vi "JSON Editor.vi"() -> ()   [LabVIEW 2024]
uses:
  WebView_class/Editor Mode--enum.ctl
  WebView.JSONEditor_class/WebView.JSONEditor.lvclass/WebView.JSONEditor.ctl
  WebView.JSONEditor_class/properties/Get JSONEditor Events.vi
  WebView.JSONEditor_class/WebView.JSONEditor.lvclass
  <vilib>/JDP Science/JSONtext/JSONtext.lvlib
  <vilib>/sklein/WebView2/Libs/Microsoft.Web.WebView2.WinForms.dll
panel:
  in  "Mode":T1
  out "Node Path":string
  out "Error Out":errorcluster
  in  "Expand all?":bool
  in  "System Load Button":bool
  in  "Stop":bool
  in  "Tab Control":enum32{"JSON", "JSON Schema"}(tab)
  in  "JSON (transparent)":string
  in  "JSON Schema":string
  in  "WebView2 Control in":refnum<k24>(container)
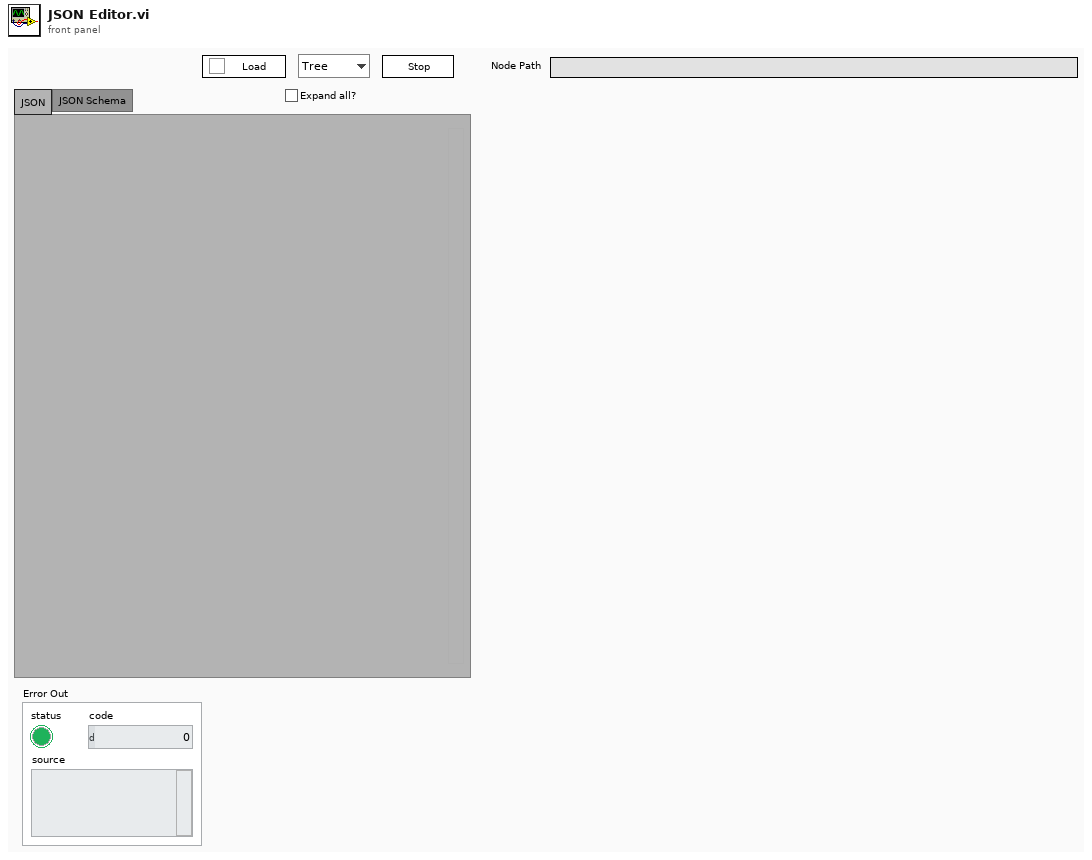
[diagram p1: front panel]
types:
  T1 = typedef "WebView.JSONEditor.lvclass/Editor Mode--enum.ctl" = enum16{"Tree", "View", "Form", "Code", "Text"}
  T2 = typedef "WebView.JSONEditor.lvclass/JSONEditor Events.ctl" = cluster{"JSON Updated":refnum<user-event>, "Selected Node Path":refnum<user-event>}
  T3 = typedef "WebView.JSONEditor.lvclass/Seleced Node Path Event Data--string.ctl" = string
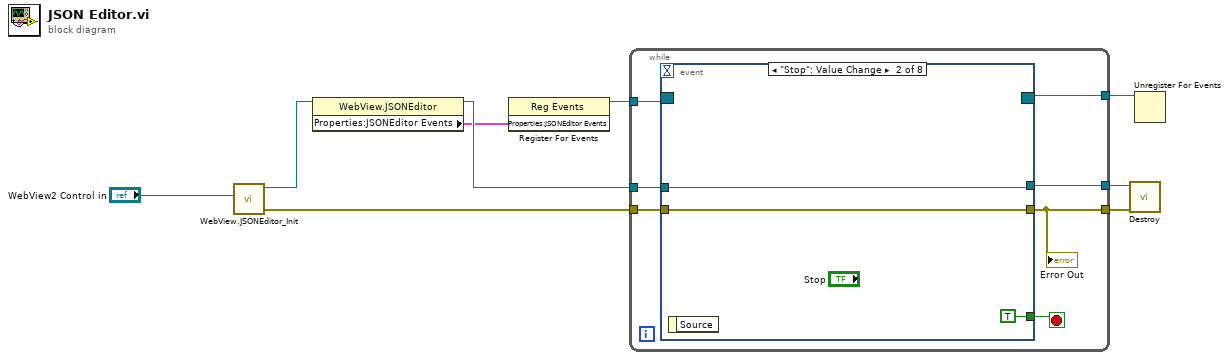
[diagram p0: block diagram]
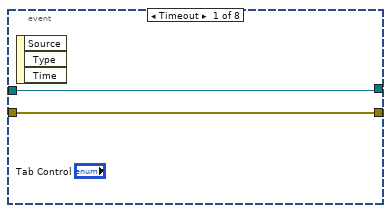
[diagram p2: hidden frame]
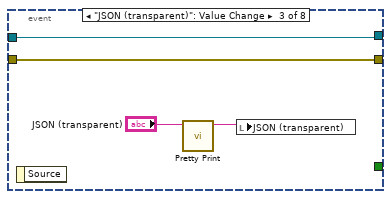
[diagram p3: hidden frame]
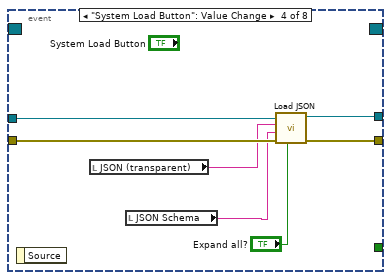
[diagram p4: hidden frame]
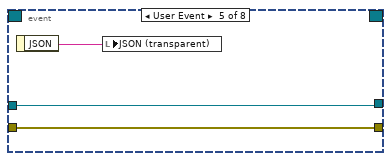
[diagram p5: hidden frame]
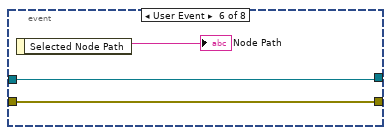
[diagram p6: hidden frame]
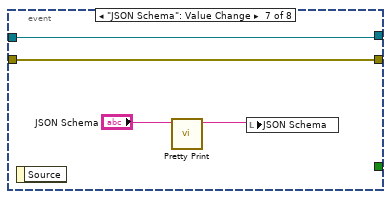
[diagram p7: hidden frame]
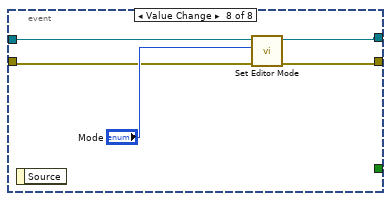
[diagram p8: hidden frame]
diagram:
  n1 = call "WebView.JSONEditor_Init.vi"("WebView2 Control in"="WebView2 Control in") -> ("Error Out"=w7:errorcluster, "WebView.JSONEditor out"=w8:refnum<class "WebView.JSONEditor.lvclass">)  [unwired: 9 in]
  n2 = property class="WebView.JSONEditor"(reference=w8) -> (reference out=w4:refnum<class "WebView.JSONEditor.lvclass">, "Properties:JSONEditor Events"=w2:T2)  [unwired: 1 in, 1 out]
  n3 = register-events(w2) -> (reference out=w3:refnum<event-registration>)  [unwired: 2 in, 1 out]
  n4 = while {
    tunnel: w4 -> [w16]
    tunnel: w7 -> [w15]
    tunnel: [w12] -> w6
    tunnel: [w14] -> w5
    tunnel: w3 -> [w11]
    tunnel: [w10] -> w1
    stop <- w13 stop-if-true
    n5 = event shown="[1] \"Stop\": Value Change" {
      selector: w11 -> [_ _ _ _ _ _ _ _]
      dyn-events: [_ _ _ _ _ _ _ _] -> w10
      timeout: _ -> [_ _ _ _ _ _ _ _]
      tunnel: w16 -> [w18 w19 w23 w31 w34 w37 w40 w46]
      tunnel: w15 -> [w17 w20 w22 w30 w35 w38 w39 w44]
      tunnel: [w17 w20 w22 w29 w35 w38 w39 w43] -> w12
      tunnel: [w18 w19 w23 w28 w34 w37 w40 w47] -> w14
      tunnel: [_ TRUE _ _ _ _ _ _] -> w13
      event Timeout {
        n6 = event-data() -> ()  [unwired: 1 in, 3 out]
      }
      event "Stop": Value Change {
        n7 = event-data() -> ()  [unwired: 1 in, 1 out]
      }
      event "JSON (transparent)": Value Change {
        n8 = event-data() -> ()  [unwired: 1 in, 1 out]
        n9 = call <vilib>:"Pretty Print.vi"("JSON"="JSON (transparent)") -> ("<JSON>"=w24:string)  [unwired: 8 in, 2 out]
        n10 = local write "JSON (transparent)"(w24) -> ()
      }
      event "System Load Button": Value Change {
        n11 = event-data() -> ()  [unwired: 1 in, 1 out]
        n12 = local read "JSON (transparent)"() -> (w27:string)
        n13 = local read "JSON Schema"() -> (w26:string)
        n14 = call "Load JSON.vi"("Expand all?"="Expand all?", "Error In"=w30, "JSON Schema in"=w26, "<JSON> in"=w27, "WebView.JSONEditor in"=w31) -> ("Error Out"=w29:errorcluster, "WebView.JSONEditor out"=w28:refnum<class "WebView.JSONEditor.lvclass">)  [unwired: 5 in]
      }
      event User Event {
        n15 = event-data() -> ("JSON"=w33:string)  [unwired: 1 in]
        n16 = local write "JSON (transparent)"(w33) -> ()
      }
      event User Event {
        n17 = event-data() -> ("Selected Node Path"=→"Node Path":T3)  [unwired: 1 in]
      }
      event "JSON Schema": Value Change {
        n18 = event-data() -> ()  [unwired: 1 in, 1 out]
        n19 = call <vilib>:"Pretty Print.vi"("JSON"="JSON Schema") -> ("<JSON>"=w41:string)  [unwired: 8 in, 2 out]
        n20 = local write "JSON Schema"(w41) -> ()
      }
      event Value Change {
        n21 = event-data() -> ()  [unwired: 1 in, 1 out]
        n22 = call-dynamic "Set Editor Mode.vi"("Error In"=w44, "Mode in"="Mode", "object in"=w46) -> ("Error Out"=w43:errorcluster, "object out"=w47:refnum<class "WebView.JSONEditor.lvclass">)  [unwired: 7 in]
      }
    }
    "Error Out" <- w12
  }
  n23 = call-dynamic "Destroy.vi"("Error In"=w6, "WebView.JSONEditor in"=w5) -> ()  [unwired: 9 in, 1 out]
  n24 = Unregister For Events(event registration refnum=w1) -> ()  [unwired: 1 in, 1 out]
